vi "Read Channel GUI Array.vi"(8 "error in (no error)":errorcluster, 11 "SPARC4_GUI in":refnum<class "S4GEI.lvclass">) -> (0 "error out":errorcluster, 2 "Channel.lvclass":refnum<class "Channel.lvclass">, 3 "SPARC4_GUI out":refnum<class "S4GEI.lvclass">)   [LabVIEW 2018, in "S4GEI.lvclass"]
uses:
  S4GEI.lvclass
  Channel GUI/Channel.lvclass
  S4GEI.lvclass/S4GEI.ctl
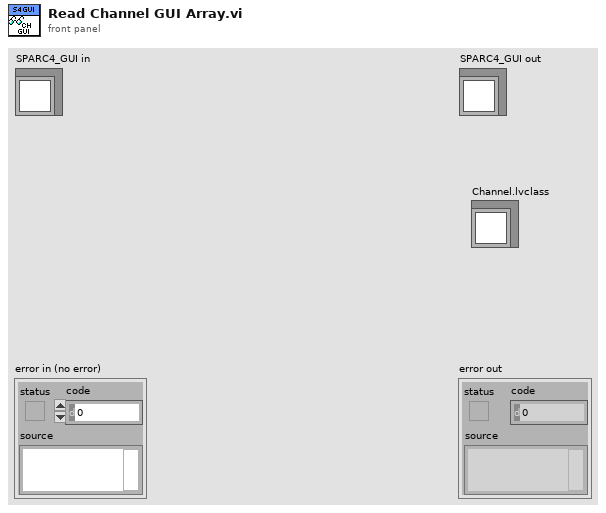
[diagram p1: front panel]
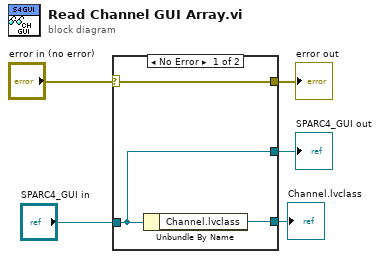
[diagram p0: block diagram]
diagram:
  n1 = case shown="No Error" "error in (no error)" {
    selector: "error in (no error)" -> [w8 w9]
    tunnel: [w8 w9] -> w4
    tunnel: [w7 w10] -> w2
    tunnel: "SPARC4_GUI in" -> [w7 w10]
    tunnel: [w6 _] -> w1
    frame No Error {
      n2 = Unbundle By Name(w7) -> ("Channel.lvclass"=w6:refnum<class "Channel.lvclass">)
    }
    frame Error {
    }
  }
  "error out" <- w4
  "SPARC4_GUI out" <- w2
  "Channel.lvclass" <- w1
